vi "killPythonServer.vi"() -> ()   [LabVIEW 2018]
panel:
  in  "error in (no error)":errorcluster
  out "error out":errorcluster
  in  "command line (built-in)":string="taskkill /IM python.exe"
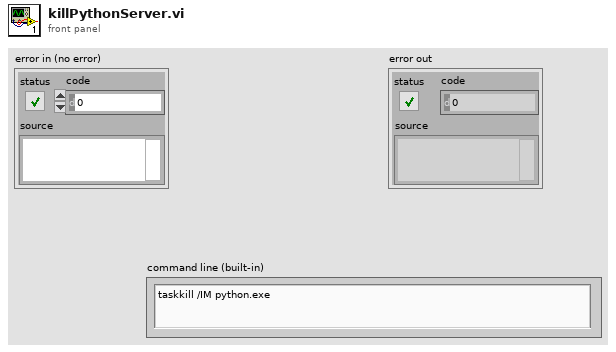
[diagram p1: front panel]
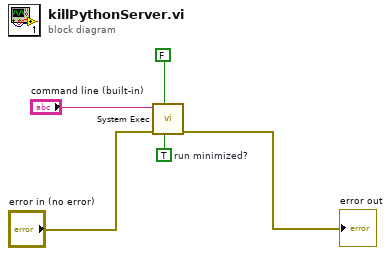
[diagram p0: block diagram]
diagram:
  w4 = TRUE  # run minimized?
  n1 = call <vilib>:"System Exec.vi"("run minimized? (F)"=w4, "wait until completion? (T)"=FALSE, "error in (no error)"="error in (no error)", "command line"="command line (built-in)") -> ("error out"=→"error out":errorcluster)  [unwired: 2 in, 5 out]
